vi "UserVars-Substitute Expression Into Expression.vi"(0 "Expression In":string, 7 "UserVars":T1[](array[typedef]), 11 "error in (no error)":errorcluster) -> (4 "Expression Out":string, 15 "error out":errorcluster)   [LabVIEW 2015]
uses:
  Tosca/LV Source/Typedefs/Tosca-Rove Variable.ctl
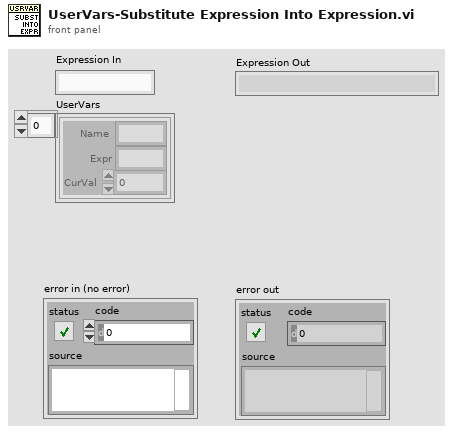
[diagram p1: front panel]
types:
  T1 = typedef "Tosca-Rove Variable.ctl" = cluster{"Name":string, "Expr":string, "CurVal":dbl}
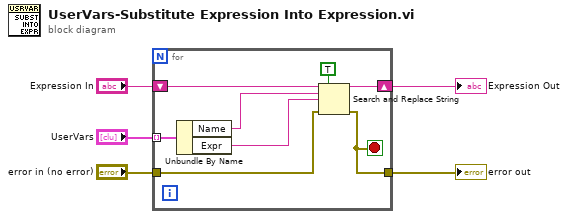
[diagram p0: block diagram]
diagram:
  n1 = for {
    tunnel: "UserVars" -> [w13] mode=indexing
    shift-right: [w10] -> w1
    shift-left: "Expression In" -> [w12]
    tunnel: "error in (no error)" -> [w8]
    tunnel: [w7] -> w2
    stop <- w7 stop-if-true
    n2 = Unbundle By Name(w13) -> ("Name"=w11:string, "Expr"=w6:string)
    n3 = Search and Replace String(replace all?=TRUE ("replace all? (F)"), input string=w12, search string=w11, replace string=w6, error in=w8) -> (result string=w10:string, error out=w7:errorcluster)  [unwired: 3 in, 2 out]
  }
  "error out" <- w2
  "Expression Out" <- w1
